vi "main_v1.vi"() -> ()   [LabVIEW 2016]
uses:
  type defs/btn_settings.ctl
panel:
  in  "Reset (\"0\")":bool
  in  "Settings":T1
  in  "Time Set(min:sec)":string caption="Thêi gian ®Æt:"
  out "Time left":string
  in  "Start":bool
  in  "Save Enable":bool caption="L­u file"
  in  "Log File":path
  in  "Stop Button":bool
  out "OK":bool
  out "NG":bool caption="OK"
  out "result":string
  out "Waveform Chart":dbl(graph) caption="BIÓU §å LùC ÐP THEO THêI GIAN"
  # "CH¦¥NG TR×NH KIÓM TRA KÝCH THñY LùC"
  # "Phßng NC MBDC - VKT"
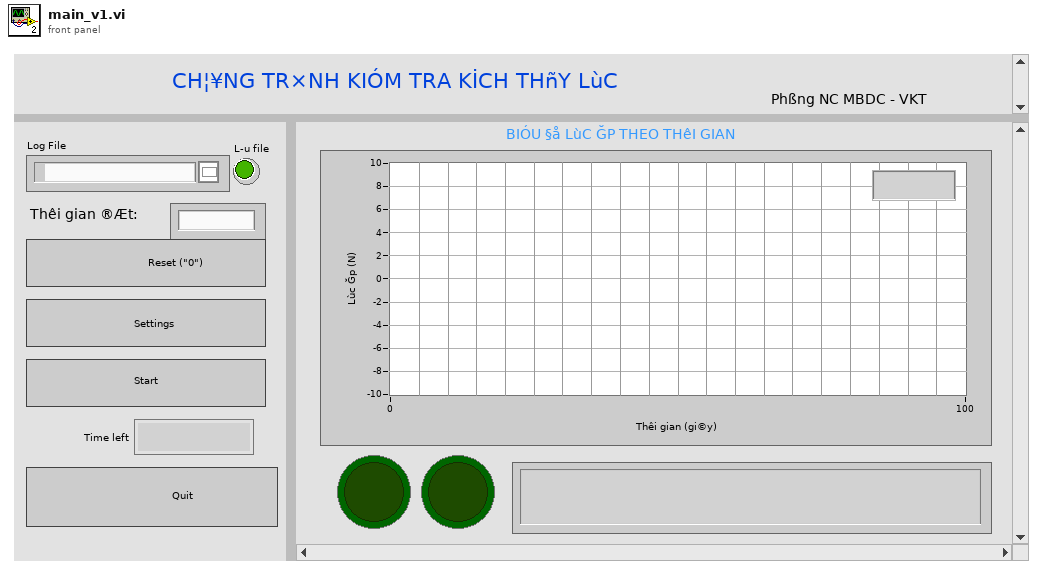
[diagram p1: front panel]
types:
  T1 = typedef "btn_settings.ctl" = bool
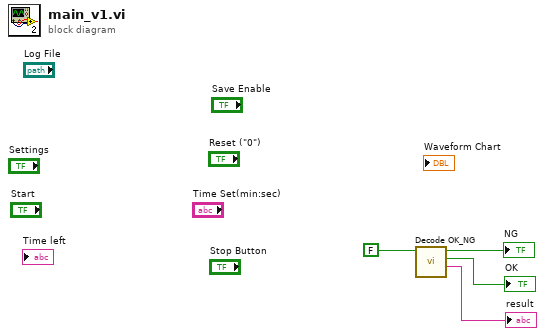
[diagram p0: block diagram]
diagram:
  n1 = call "Decode OK_NG.vi"("Boolean"=FALSE) -> ("result"=→"result":string, "OK"=→"OK":bool, "NG"=→"NG":bool)  [unwired: 8 in]
